vi "ListIO.vi"(11 "Project":refnum<vi>) -> (0 "DI/O":string[](array[string]), 1 "AI":string[](array[string]), 2 "AO":string[](array[string]), 3 "DIOPORT":string[](array[string]))   [LabVIEW 2023]
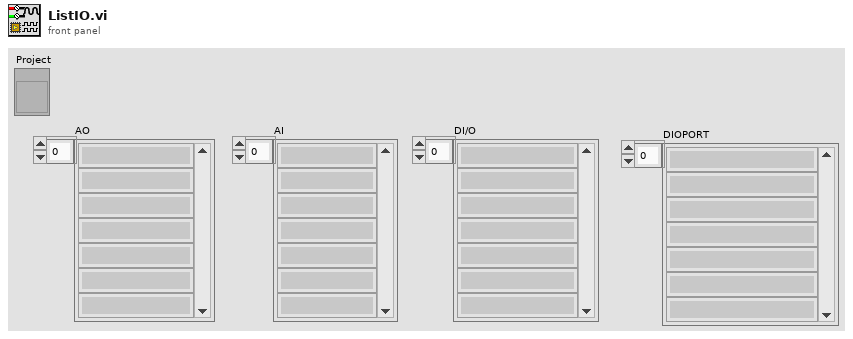
[diagram p1: front panel]
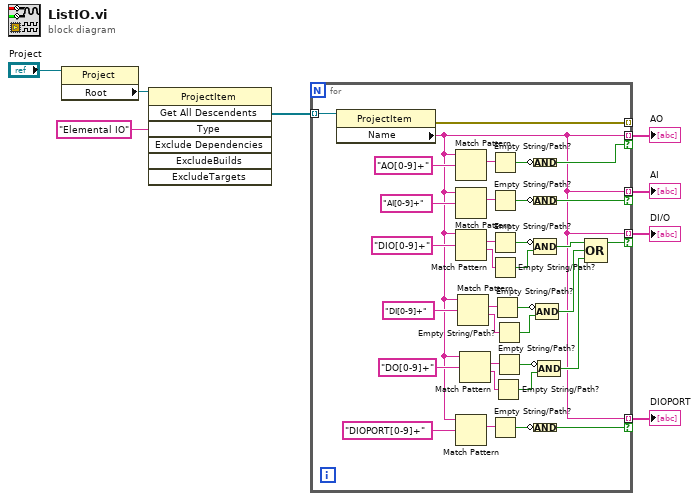
[diagram p0: block diagram]
diagram:
  n1 = property class="Project"(reference="Project") -> ("Root"=w6:refnum<vi>)  [unwired: 1 in, 2 out]
  n2 = invoke class="ProjectItem" method="Get All Descendents"(reference=w6, "Type"="Elemental IO" ("Type String")) -> ("All Descendents"=w7:refnum<vi>[])  [unwired: 5 in, 6 out]
  n3 = for {
    tunnel: w7 -> [w42] mode=indexing
    tunnel: [w15] -> w8 mode=indexing if=w38
    tunnel: [w41] -> _ mode=indexing
    tunnel: [w15] -> w4 mode=indexing if=w30
    tunnel: [w15] -> w3 mode=indexing if=w21
    tunnel: [w15] -> w1 mode=indexing if=w25
    n4 = property class="ProjectItem"(reference=w42) -> (error out=w41:errorcluster, "Name"=w15:string)  [unwired: 1 in, 1 out]
    n5 = Match Pattern(string=w15, regular expression="AO[0-9]+") -> (match substring=w39:string)  [unwired: 1 in, 3 out]
    n6 = Match Pattern(string=w15, regular expression="AI[0-9]+") -> (match substring=w35:string)  [unwired: 1 in, 3 out]
    n7 = Match Pattern(string=w15, regular expression="DIO[0-9]+") -> (match substring=w32:string, after substring=w10:string)  [unwired: 1 in, 2 out]
    n8 = Match Pattern(string=w15, regular expression="DIOPORT[0-9]+") -> (match substring=w27:string)  [unwired: 1 in, 3 out]
    n9 = Match Pattern(string=w15, regular expression="DI[0-9]+") -> (match substring=w23:string, after substring=w11:string)  [unwired: 1 in, 2 out]
    n10 = Match Pattern(string=w15, regular expression="DO[0-9]+") -> (match substring=w18:string, after substring=w14:string)  [unwired: 1 in, 2 out]
    n11 = Empty String/Path?(string/path=w39) -> (empty?=w37:bool)
    n12 = Empty String/Path?(string/path=w35) -> (empty?=w36:bool)
    n13 = Empty String/Path?(string/path=w32) -> (empty?=w31:bool)
    n14 = Empty String/Path?(string/path=w10) -> (empty?=w9:bool)
    n15 = Empty String/Path?(string/path=w27) -> (empty?=w28:bool)
    n16 = Empty String/Path?(string/path=w23) -> (empty?=w24:bool)
    n17 = Empty String/Path?(string/path=w14) -> (empty?=w13:bool)
    n18 = Empty String/Path?(string/path=w11) -> (empty?=w12:bool)
    n19 = Empty String/Path?(string/path=w18) -> (empty?=w17:bool)
    n20 = Compound Arithmetic op=AND(invert w37) -> (w38:bool)
    n21 = Compound Arithmetic op=AND(invert w36) -> (w30:bool)
    n22 = Compound Arithmetic op=AND(invert w31, w9) -> (w29:bool)
    n23 = Compound Arithmetic op=AND(invert w28) -> (w25:bool)
    n24 = Compound Arithmetic op=AND(invert w24, w12) -> (w20:bool)
    n25 = Compound Arithmetic op=AND(invert w17, w13) -> (w16:bool)
    n26 = Compound Arithmetic op=OR(w29, w20, w16) -> (w21:bool)
  }
  "AO" <- w8
  "AI" <- w4
  "DI/O" <- w3
  "DIOPORT" <- w1
